vi "Runner.vi"() -> ()   [LabVIEW 2021]
uses:
  <vilib>/Hampel Software Engineering/Git API/Git API/GIT-api.lvclass/GIT-api.ctl
  0bad4ac3-91b5-4d0e-a986-299fb1bc9cfd.vi
  <vilib>/Hampel Software Engineering/Git API/Git API/Accessors/GIT-Set Working Dir.vi
  <vilib>/Hampel Software Engineering/Git API/Git API/GIT-api.lvclass
panel:
  out "Numeric":i32
  out "error out":errorcluster
  in  "stop":bool
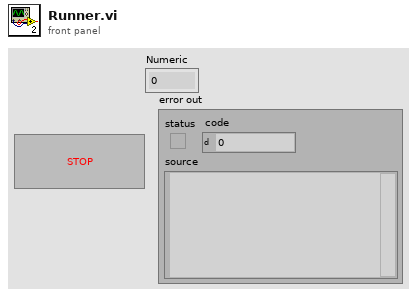
[diagram p1: front panel]
types:
  T1 = typedef "GIT-API-for-LabVIEW.lvlib/GIT-api.lvclass/GIT-Repository States.ctl" = enum16{"up-to-date", "behind", "ahead", "diverged", "unpublished", "detached", "unknown"}
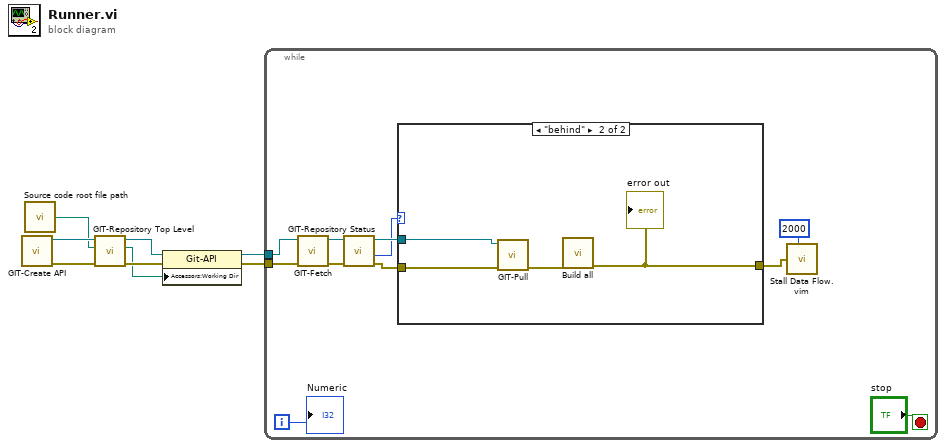
[diagram p0: block diagram]
diagram:
  n1 = call <vilib>:"GIT-Create API.vi"() -> ("error out"=w5:errorcluster, "git-api out"=w7:refnum<class "GIT-api.lvclass">)  [unwired: 10 in]
  n2 = call "Source code root file path.vi"() -> ("Source code root path"=w4:path)  [unwired: 1 in]
  n3 = call <vilib>:"GIT-Repository Top Level.vi"("error in"=w5, "Current Path"=w4, "git-api in"=w7) -> ("error out"=w6:errorcluster, "Repo Top Level Path"=w3:path, "git-api out"=w8:refnum<class "GIT-api.lvclass">)  [unwired: 6 in]
  n4 = property class="Git-API"(reference=w8, error in=w6, "Accessors:Working Dir"=w3) -> (reference out=w1:refnum<class "GIT-api.lvclass">, error out=w2:errorcluster)
  n5 = while {
    tunnel: w2 -> [w10]
    tunnel: w1 -> [w9]
    i -> [w13]
    stop <- "stop" stop-if-true
    n6 = call <vilib>:"GIT-Fetch.vi"("error in"=w10, "git-api in"=w9) -> ("error out"=w11:errorcluster, "git-api out"=w12:refnum<class "GIT-api.lvclass">)  [unwired: 7 in, 1 out]
    n7 = call <vilib>:"GIT-Repository Status.vi"("error in"=w11, "git-api in"=w12) -> ("error out"=w18:errorcluster, "State"=w16:T1, "git-api out"=w17:refnum<class "GIT-api.lvclass">)  [unwired: 6 in, 1 out]
    n8 = case shown="\"behind\"" w16 {
      tunnel: w18 -> [_ w21]
      tunnel: w17 -> [_ w20]
      tunnel: [_ w22] -> w15
      frame "up-to-date", Default {
      }
      frame "behind" {
        n9 = call <vilib>:"GIT-Pull.vi"("error in"=w21, "git-api in"=w20) -> ("error out"=w23:errorcluster)  [unwired: 8 in, 1 out]
        n10 = call "Build all.vi"("error in (no error)"=w23) -> ("error out"=w22:errorcluster)  [unwired: 10 in]
        "error out" <- w22
      }
    }
    n11 = call "Stall Data Flow.vim"("value in"=w15, "milliseconds to wait"=u32 2000) -> ()  [unwired: 2 out]
    "Numeric" <- w13
  }
